vi "HEXandASCIIConverter.vi"(9 "ASCII 格式輸入":string, 10 "HEX 格式輸入":string) -> (2 "16進制格式輸出":string, 3 "ASCII 格式輸出":string)   [LabVIEW 2019]
panel:
  out "十進位數值輸出":u8
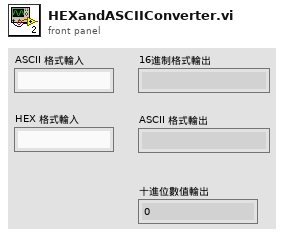
[diagram p1: front panel]
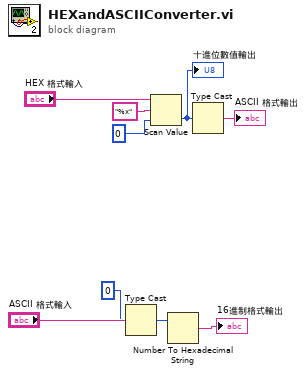
[diagram p0: block diagram]
diagram:
  n1 = Type Cast(type=u8 0 ("Decimal value"), x="ASCII 格式輸入") -> (*(type *) &x=w8:u8)
  n2 = Scan Value(string="HEX 格式輸入", format string="%x", default (0 dbl)=u8 0 ("number")) -> (value=w7:u8)  [unwired: 1 out]
  "十進位數值輸出" <- w7
  n3 = Number To Hexadecimal String(2:w8) -> (0:→"16進制格式輸出":string)  [unwired: 1 out]
  n4 = Type Cast(x=w7) -> (*(type *) &x=→"ASCII 格式輸出":string)  [unwired: 1 out]
